vi "Audio_Transformation_Setted_Frequency_v006.vi"() -> ()   [LabVIEW 2019]
uses:
  <vilib>/addons/_Advanced Signal Processing/NI_AdvSigProcTFA.lvlib
  <vilib>/sound2/lvsound2.llb/Sound Data Format.ctl
  <vilib>/sound2/lvsound2.llb/Sound Input Read (DBL).vi
  <vilib>/addons/Time Frequency Analysis/Transform.llb/TFA Online Gabor Transform (Real).vi
panel:
  out "u(t)":T1(graph)
  out "V(t)":T1(graph)
  out "Noise Speech":dbl[](graph)
  in  "Address selector":i32[](array[numeric])
  in  "Neuron Type":T2(ring)
  out "max index(es)":i32
  out "max value":dbl
  out "Waveform Graph":dbl[](graph)
  out "Magnitude of Gabor Coefficients":dbl[][](graph)
  in  "Stop":bool
  # "Step two : Graph of the amplitude of the Gabor coefficient of the different bins"
  # "Step three : Spike Response of the neurons"
  # "Step one: Sound recorded from the computer"
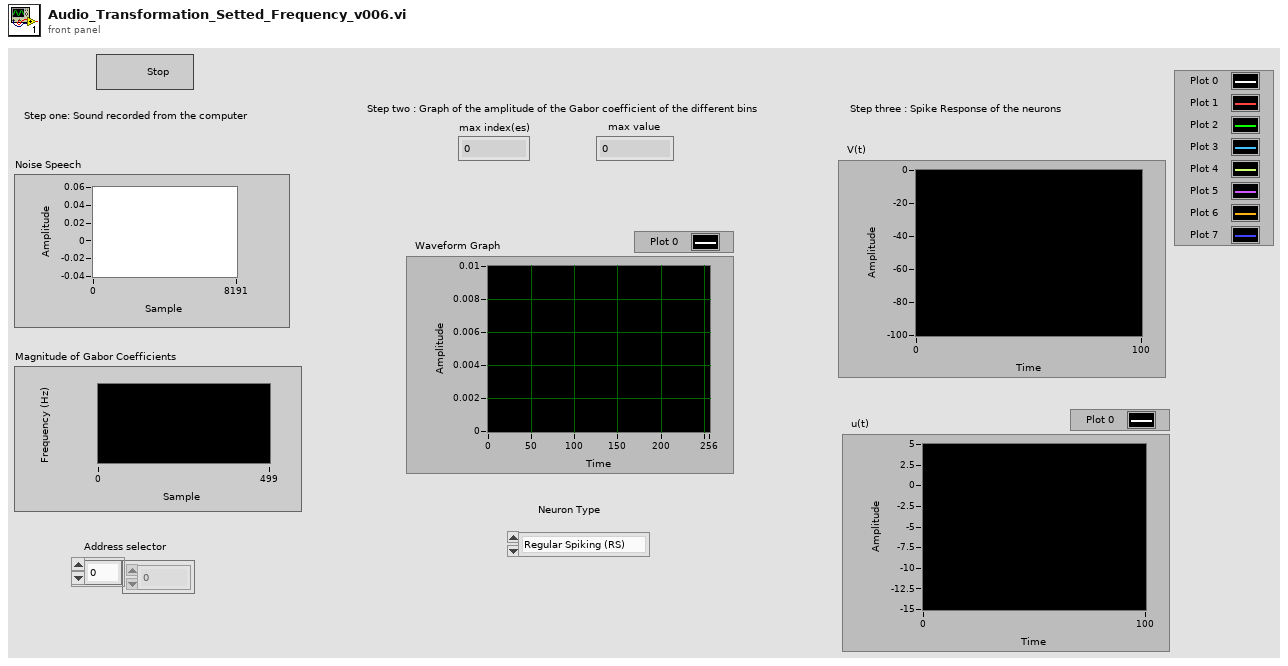
[diagram p1: front panel]
types:
  T1 = cluster{"[0]":dbl, "[1]":dbl, "[2]":dbl, "[3]":dbl, "[4]":dbl, "[5]":dbl, "[6]":dbl, "[7]":dbl, "[8]":dbl}
  T2 = enum16{"Regular Spiking (RS)", "Intrinsically Bursting (IB)", "Chattering (CH)", "Fast Spiking (FS)", "Thalamo-Cortical 1 (TC1)", "Thalamo-Cortical 2 (TC2)", "Resonator (RZ)", "Low-Threshold Spiking (LTS)"}
  T3 = typedef "Sound Data Format.ctl" = cluster{"sample rate (S/s)":dbl, "number of channels":i32, "bits per sample":i32}
  T4 = typedef "Sound Input Task ID.ctl" = u32
  T5 = cluster{"analysis window":dbl[], "dM (time steps)":i32, "N (frequency bins)":i32}
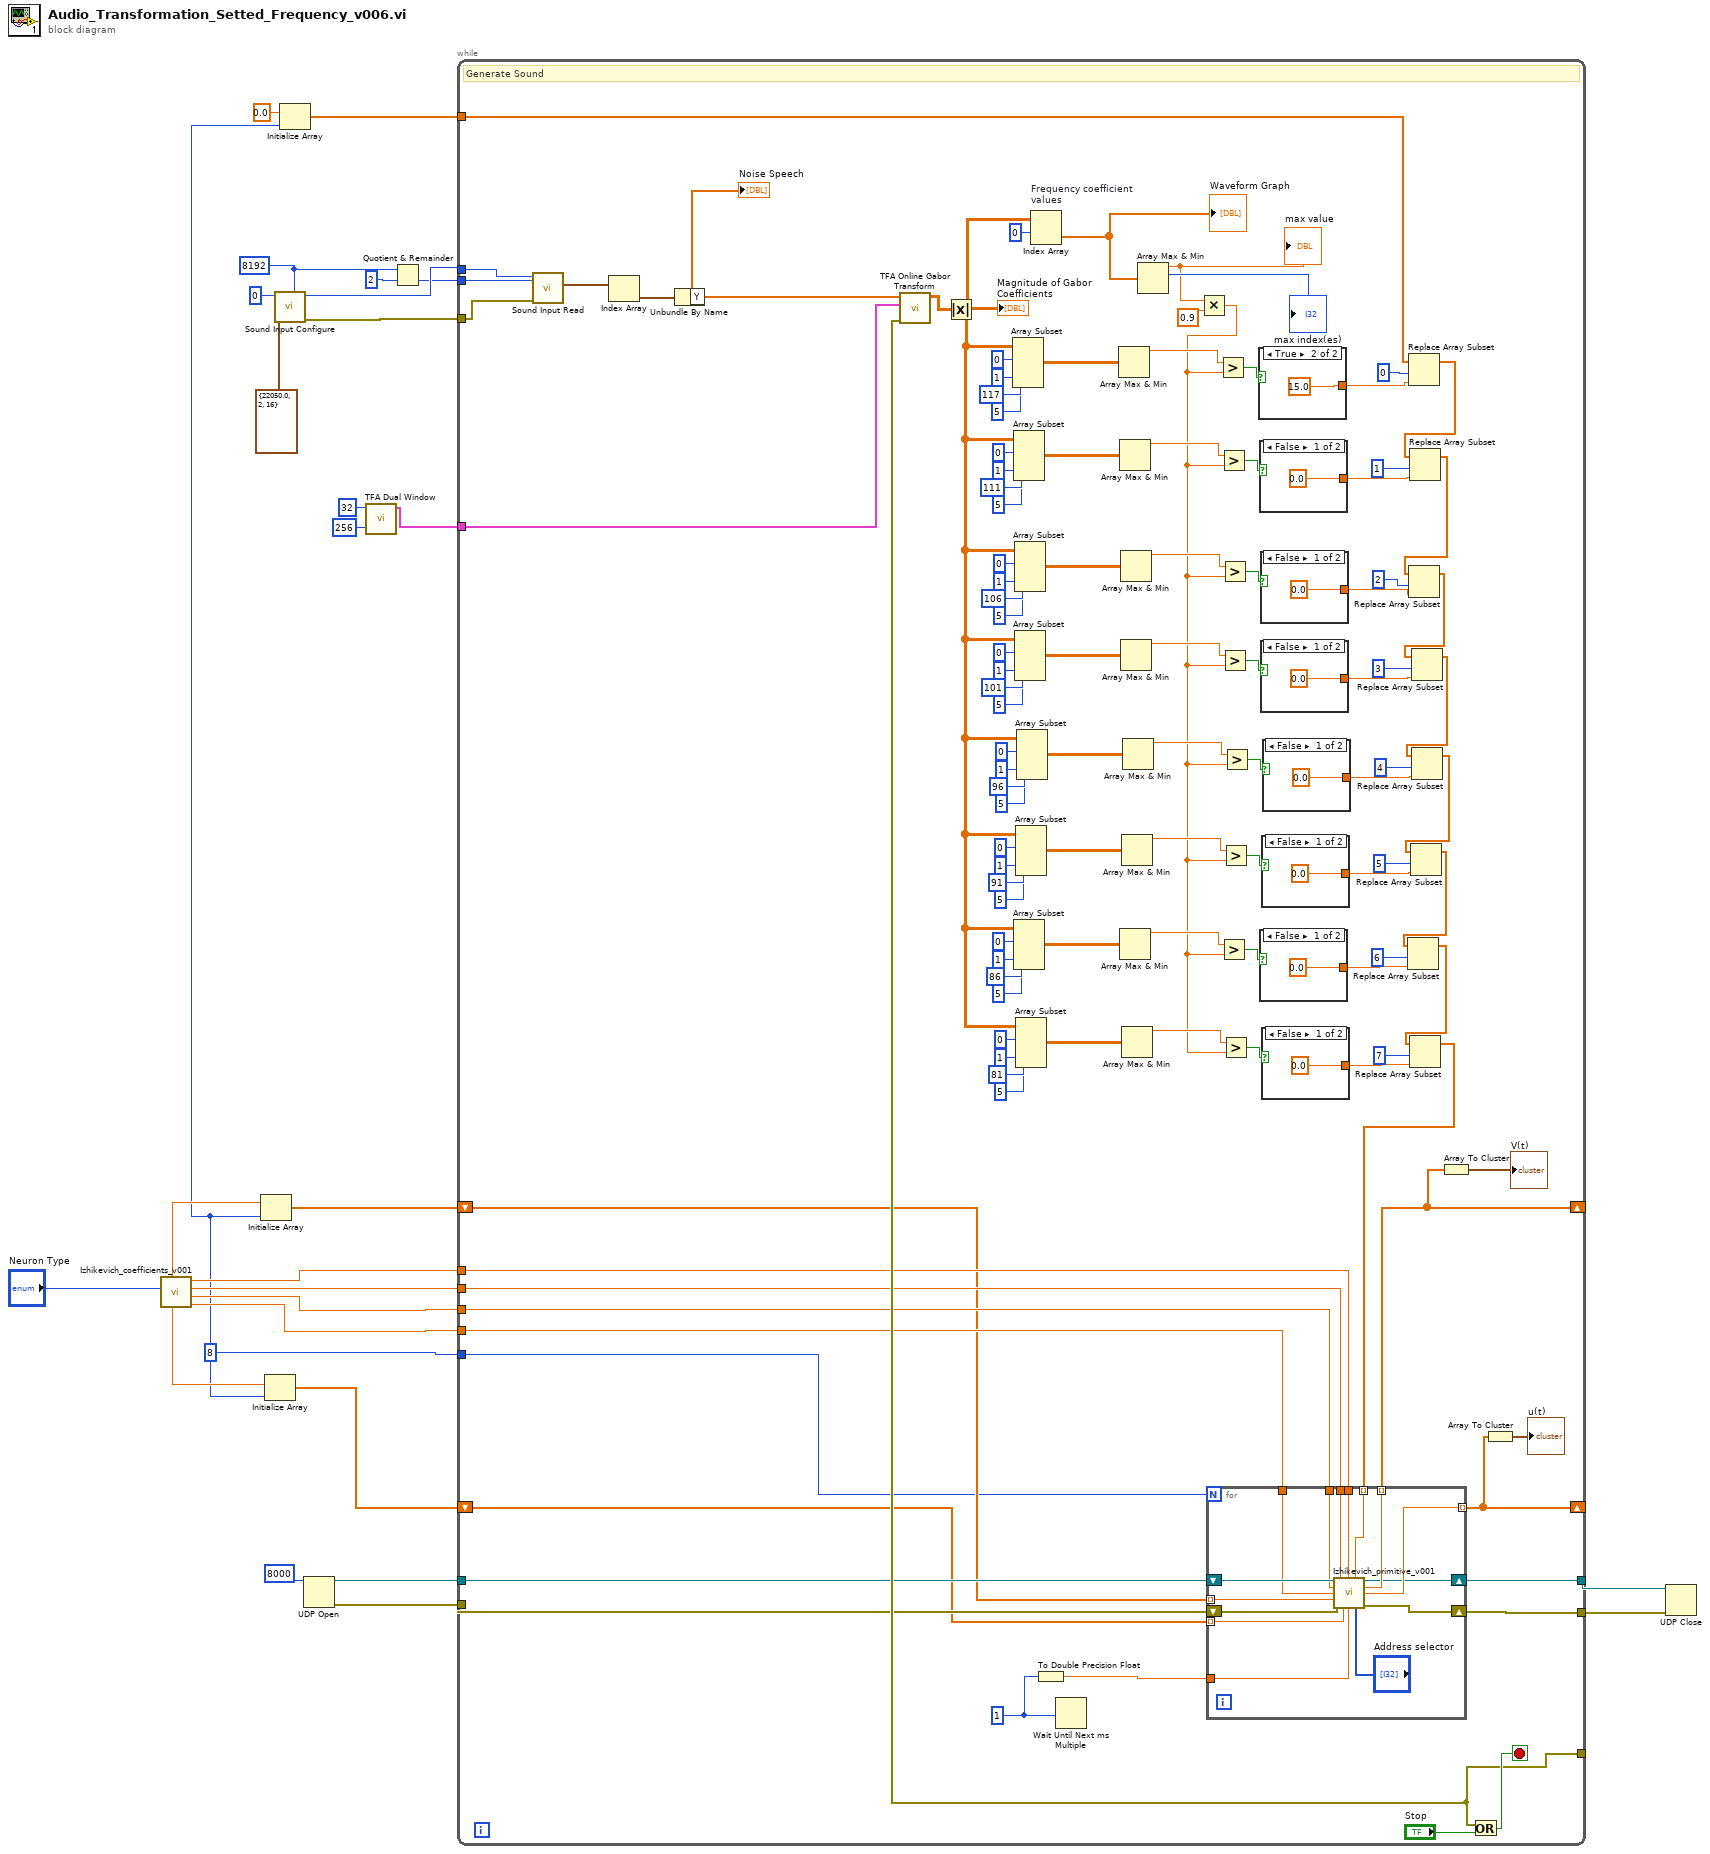
[diagram p0: block diagram]
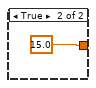
[diagram p2: hidden frame]
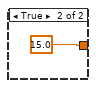
[diagram p3: hidden frame]
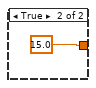
[diagram p4: hidden frame]
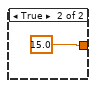
[diagram p5: hidden frame]
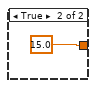
[diagram p6: hidden frame]
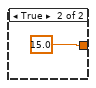
[diagram p7: hidden frame]
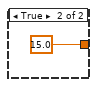
[diagram p8: hidden frame]
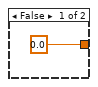
[diagram p9: hidden frame]
diagram:
  w3 = 8
  w12 = 8192 ("number of samples/ch")
  n1 = call "Izhikevich_coefficients_v001.vi"("Neuron Type"="Neuron Type") -> ("d"=w20:dbl, "c"=w21:dbl, "b"=w22:dbl, "a"=w23:dbl, "u0"=w5:dbl, "v0"=w7:dbl)  [unwired: 3 in]
  n2 = Initialize Array(w7, w3) -> (w6:dbl[])
  n3 = Initialize Array(w5, w3) -> (w4:dbl[])
  n4 = call <vilib>:"Sound Input Configure.vi"("number of samples/ch"=w12, "sound format"=T3 {"sample rate (S/s)"=22050.0, "number of channels"=2, "bits per sample"=16}, "device ID"=u32 0) -> ("error out"=w9:errorcluster, "task ID"=w10:T4)  [unwired: 7 in]
  n5 = Initialize Array(0.0 ("element"), w3) -> (w1:dbl[])
  n6 = UDP Open(11:u16 8000 ("port")) -> (port=w18:refnum<k16>, 0:w17:errorcluster)  [unwired: 4 in, 1 out]
  n7 = call <vilib>:"TFA Dual Window.vi"("N (frequency bins)"=256, "dM (time steps)"=32) -> ("analysis info"=w25:T5)  [unwired: 7 in, 2 out]
  n8 = Quotient & Remainder(x=w12, y=2) -> (floor(x/y)=w8:i32)  [unwired: 1 out]
  n9 = while {
    tunnel: [w136] -> _
    tunnel: w25 -> [w141]
    shift-right: [w32] -> _
    shift-left: w6 -> [w125]
    shift-right: [w30] -> _
    shift-left: w4 -> [w124]
    tunnel: w23 -> [w135]
    tunnel: w22 -> [w134]
    tunnel: w21 -> [w132]
    tunnel: w20 -> [w131]
    tunnel: w18 -> [w133]
    tunnel: w17 -> [w130]
    tunnel: [w127] -> w16
    tunnel: [w126] -> w15
    tunnel: w10 -> [w122]
    tunnel: w9 -> [w121]
    tunnel: w8 -> [w123]
    tunnel: w3 -> [w117]
    tunnel: w1 -> [w88]
    stop <- w142 stop-if-true
    w129 = u32 1 ("millisecond multiple")
    # "Generate Sound"
    n10 = call-poly <vilib>:"Sound Input Read.vi"("number of samples/ch"=w123, "error in (no error)"=w121, "task ID"=w122) -> ("data"=w119:waveform(dbl)[])  [unwired: 6 in, 2 out]
    n11 = Index Array(array=w119) -> (element=w120:waveform(dbl))  [unwired: 1 in]
    n12 = Unbundle By Name(w120) -> ("Y"=w118:dbl[])
    "Noise Speech" <- w118
    n13 = call-poly <vilib>:"TFA Online Gabor Transform.vi"("transform info"=w141, "signal"=w118) -> ("error out"=w136:errorcluster, "Gabor coef"=w140:cdb[][])  [unwired: 7 in, 1 out]
    n14 = Absolute Value(x=w140) -> (abs(x)=w36:dbl[][])
    "Magnitude of Gabor Coefficients" <- w36
    n15 = Array Subset(array=w36, index (row)=0 ("index"), length (row)=1 ("length"), index (col)=117 ("index"), length (col)=5 ("length")) -> (w112:dbl[][])
    n16 = Array Subset(array=w36, index (row)=0 ("index"), length (row)=1 ("length"), index (col)=111 ("index"), length (col)=5 ("length")) -> (w104:dbl[][])
    n17 = Array Subset(array=w36, index (row)=0 ("index"), length (row)=1 ("length"), index (col)=86 ("index"), length (col)=5 ("length")) -> (w51:dbl[][])
    n18 = Array Subset(array=w36, index (row)=0 ("index"), length (row)=1 ("length"), index (col)=106 ("index"), length (col)=5 ("length")) -> (w93:dbl[][])
    n19 = Array Subset(array=w36, index (row)=0 ("index"), length (row)=1 ("length"), index (col)=101 ("index"), length (col)=5 ("length")) -> (w81:dbl[][])
    n20 = Array Subset(array=w36, index (row)=0 ("index"), length (row)=1 ("length"), index (col)=91 ("index"), length (col)=5 ("length")) -> (w61:dbl[][])
    n21 = Array Subset(array=w36, index (row)=0 ("index"), length (row)=1 ("length"), index (col)=81 ("index"), length (col)=5 ("length")) -> (w41:dbl[][])
    n22 = Array Subset(array=w36, index (row)=0 ("index"), length (row)=1 ("length"), index (col)=96 ("index"), length (col)=5 ("length")) -> (w71:dbl[][])
    n23 = Index Array "Frequency coefficient \nvalues"(array=w36, index (row)=0) -> (element=w138:dbl[])  [unwired: 1 in]
    "Waveform Graph" <- w138
    n24 = To Double Precision Float(number=w129) -> (double precision float=w128:dbl)
    n25 = Wait Until Next ms Multiple(millisecond multiple=w129) -> ()  [unwired: 1 out]
    n26 = Array Max & Min(array=w112) -> (max value=w110:dbl)  [unwired: 3 out]
    n27 = Array Max & Min(array=w104) -> (max value=w103:dbl)  [unwired: 3 out]
    n28 = Array Max & Min(array=w51) -> (max value=w50:dbl)  [unwired: 3 out]
    n29 = Array Max & Min(array=w93) -> (max value=w92:dbl)  [unwired: 3 out]
    n30 = Array Max & Min(array=w81) -> (max value=w80:dbl)  [unwired: 3 out]
    n31 = Array Max & Min(array=w61) -> (max value=w60:dbl)  [unwired: 3 out]
    n32 = Array Max & Min(array=w41) -> (max value=w40:dbl)  [unwired: 3 out]
    n33 = Array Max & Min(array=w71) -> (max value=w70:dbl)  [unwired: 3 out]
    n34 = Array Max & Min(array=w138) -> (max value=w111:dbl, max index (indices)=→"max index(es)":i32)  [unwired: 2 out]
    "max value" <- w111
    n35 = Multiply(x=w111, y=0.9) -> (x*y=w28:dbl)
    n36 = Greater?(x=w110, y=w28) -> (0:w109:bool)
    n37 = Greater?(x=w103, y=w28) -> (0:w102:bool)
    n38 = Greater?(x=w50, y=w28) -> (0:w49:bool)
    n39 = Greater?(x=w92, y=w28) -> (0:w91:bool)
    n40 = Greater?(x=w80, y=w28) -> (0:w79:bool)
    n41 = Greater?(x=w60, y=w28) -> (0:w59:bool)
    n42 = Greater?(x=w40, y=w28) -> (0:w39:bool)
    n43 = Greater?(x=w70, y=w28) -> (0:w69:bool)
    n44 = case shown="True" w109 {
      tunnel: [0.0 15.0] -> w101
      frame False {
      }
      frame True {
      }
    }
    n45 = case shown="False" w102 {
      tunnel: [0.0 15.0] -> w98
      frame False {
      }
      frame True {
      }
    }
    n46 = case shown="False" w49 {
      tunnel: [0.0 15.0] -> w47
      frame False {
      }
      frame True {
      }
    }
    n47 = case shown="False" w91 {
      tunnel: [0.0 15.0] -> w89
      frame False {
      }
      frame True {
      }
    }
    n48 = case shown="False" w79 {
      tunnel: [0.0 15.0] -> w77
      frame False {
      }
      frame True {
      }
    }
    n49 = case shown="False" w59 {
      tunnel: [0.0 15.0] -> w57
      frame False {
      }
      frame True {
      }
    }
    n50 = case shown="False" w39 {
      tunnel: [0.0 15.0] -> w37
      frame False {
      }
      frame True {
      }
    }
    n51 = case shown="False" w69 {
      tunnel: [0.0 15.0] -> w67
      frame False {
      }
      frame True {
      }
    }
    n52 = Replace Array Subset(array=w88, new element=w101, index=0) -> (w87:dbl[])
    n53 = Replace Array Subset(array=w87, new element=w98, index=1) -> (w86:dbl[])
    n54 = Replace Array Subset(array=w86, new element=w89, index=2) -> (w76:dbl[])
    n55 = Replace Array Subset(array=w76, new element=w77, index=3) -> (w66:dbl[])
    n56 = Replace Array Subset(array=w66, new element=w67, index=4) -> (w56:dbl[])
    n57 = Replace Array Subset(array=w56, new element=w57, index=5) -> (w46:dbl[])
    n58 = Replace Array Subset(array=w46, new element=w47, index=6) -> (w34:dbl[])
    n59 = Replace Array Subset(array=w34, new element=w37, index=7) -> (w33:dbl[])
    n60 = for {
      N: w117 -> [_]
      tunnel: w135 -> [w174]
      tunnel: w134 -> [w173]
      tunnel: w132 -> [w171]
      tunnel: w131 -> [w170]
      tunnel: w128 -> [w167]
      tunnel: [w166] -> w32 mode=indexing
      tunnel: [w165] -> w30 mode=indexing
      tunnel: w125 -> [w162] mode=indexing
      tunnel: w124 -> [w161] mode=indexing
      shift-right: [w163] -> w126
      shift-left: w133 -> [w172]
      shift-right: [w164] -> w127
      shift-left: w130 -> [w169]
      tunnel: w33 -> [w160] mode=indexing
      n61 = call "Izhikevich_primitive_v001.vi"("UDP Network Connection in"=w172, "b"=w173, "a"=w174, "I"=w160, "c"=w171, "d"=w170, "v(t)"=w162, "error in (no error)"=w169, "u(t)"=w161, "Numeric"=w167, "Address selector"="Address selector") -> ("UDP Network Connection out"=w163:refnum<k16>, "v(t+dt)"=w166:dbl, "u(t+dt)"=w165:dbl, "error out"=w164:errorcluster)  [unwired: 1 in]
    }
    n62 = Array To Cluster(array=w32) -> (cluster=→"V(t)":T1)
    n63 = Or(x=w136, y="Stop") -> (x .or. y?=w142:bool)
    n64 = Array To Cluster(array=w30) -> (cluster=→"u(t)":T1)
  }
  n65 = UDP Close(connection ID=w15, 8:w16) -> ()  [unwired: 2 out]
